vi "2D_Position Graphs.vi"() -> ()   [LabVIEW 2018]
panel:
  in  "velocity":dbl
  out "Z vs. t":cluster{dbl[], dbl[]}(graph)
  out "Y vs. t":cluster{dbl[], dbl[]}(graph)
  out "X vs. t":cluster{dbl[], dbl[]}(graph)
  out "zPosition":dbl
  out "xPosition":dbl
  out "vZfinal":dbl
  out "vXfinal":dbl
  out "vZinitial":dbl
  out "vXinitial":dbl
  out "vYfinal":dbl
  out "yPosition":dbl
  out "timeOfFlight":dbl format="%#_5g"
  in  "height":dbl
  out "vYinitial":dbl
  in  "eField":dbl
  in  "bField":dbl
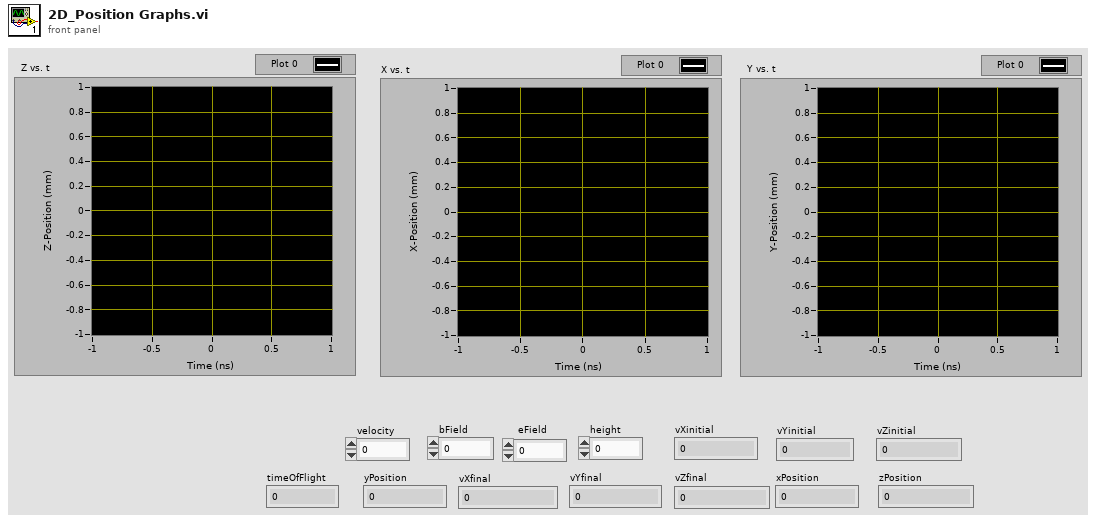
[diagram p1: front panel]
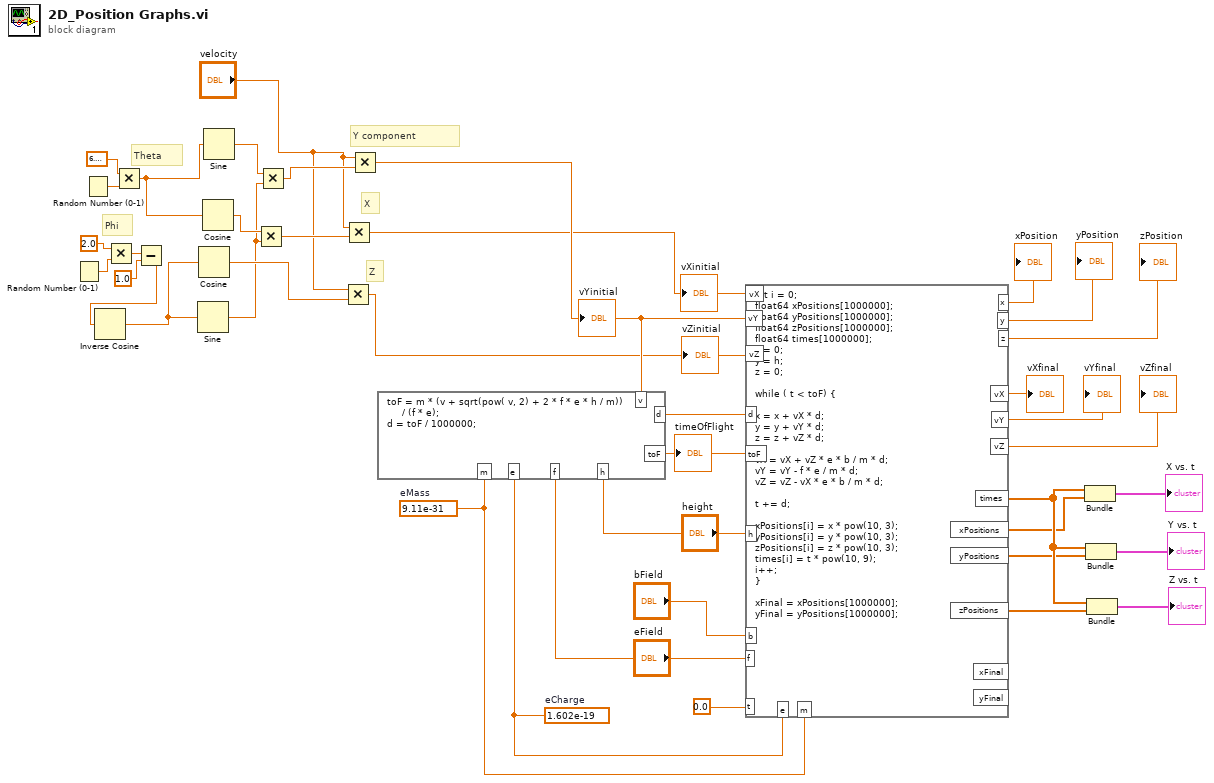
[diagram p0: block diagram]
diagram:
  w38 = 1.602e-19  # eCharge
  w37 = 9.11e-31  # eMass
  # "Phi"
  # "Theta"
  # "Z"
  # "X"
  # "Y component"
  n1 = Random Number (0-1)() -> (number: 0 to 1=w16:dbl)
  n2 = Random Number (0-1)() -> (number: 0 to 1=w19:dbl)
  n3 = Multiply(x=2.0, y=w16) -> (x*y=w15:dbl)
  n4 = Multiply(x=6.283185307179586, y=w19) -> (x*y=w13:dbl)
  n5 = Subtract(x=w15, y=1.0) -> (x-y=w12:dbl)
  n6 = Inverse Cosine(1:w12) -> (0:w11:dbl)
  n7 = Sine(x=w11) -> (sin(x)=w6:dbl)
  n8 = Cosine(x=w11) -> (cos(x)=w10:dbl)
  n9 = Cosine(x=w13) -> (cos(x)=w7:dbl)
  n10 = Sine(x=w13) -> (sin(x)=w9:dbl)
  n11 = Multiply(x=w7, y=w6) -> (x*y=w5:dbl)
  n12 = Multiply(x=w9, y=w6) -> (x*y=w8:dbl)
  n13 = Multiply(x="velocity", y=w10) -> (x*y=w2:dbl)
  "vZinitial" <- w2
  n14 = Multiply(x="velocity", y=w5) -> (x*y=w3:dbl)
  "vXinitial" <- w3
  n15 = Multiply(x="velocity", y=w8) -> (x*y=w4:dbl)
  "vYinitial" <- w4
  n16 = formula code="toF = m * (v + sqrt(pow( v, 2) + 2 * f * e * h / m))\n     / (f * e);\nd = toF / 1000000;"("f"="eField", "h"="height", "v"=w4, "m"=w37, "e"=w38) -> ("toF"=w35:dbl, "d"=w36:dbl)
  "timeOfFlight" <- w35
  n17 = formula code="int i = 0;\nfloat64 xPositions[1000000];\nfloat64 yPositions[1000000];\nfloat64 zPositions[1000000];\nfloat64 times[1000000];\nx = 0;\ny = h;\nz = 0;\n\nwhile ( t < toF) {\n\nx = x + vX * d;\ny = y + vY * d;\nz = z + vZ * d;\n\nvX = vX + vZ * e * b / m * d;\nvY = vY - f * e / m * d;\nvZ = vZ - vX * e * b / m * d;\n\nt += d;\n\nxPositions[i] = x * pow(10, 3);\nyPositions[i] = y * pow(10, 3);\nzPositions[i] = z * pow(10, 3);\ntimes[i] = t * pow(10, 9);\ni++;\n}\n\nxFinal = xPositions[1000000];\nyFinal = yPositions[1000000];"("vY"=w4, "e"=w38, "m"=w37, "f"="eField", "d"=w36, "h"="height", "toF"=w35, "t"=0.0, "b"="bField", "vX"=w3, "vZ"=w2) -> ("y"=→"yPosition":dbl, "vY"=→"vYfinal":dbl, "vX"=→"vXfinal":dbl, "vZ"=→"vZfinal":dbl, "x"=→"xPosition":dbl, "z"=→"zPosition":dbl, "xPositions"=w20:dbl[], "yPositions"=w22:dbl[], "zPositions"=w21:dbl[], "times"=w23:dbl[])  [unwired: 2 out]
  n18 = Bundle(w23, w20) -> (→"X vs. t":cluster{dbl[], dbl[]})  [unwired: 1 in]
  n19 = Bundle(w23, w22) -> (→"Y vs. t":cluster{dbl[], dbl[]})  [unwired: 1 in]
  n20 = Bundle(w23, w21) -> (→"Z vs. t":cluster{dbl[], dbl[]})  [unwired: 1 in]
